vi "GetFootnoteReference.vi"(8 "error in (no error)":errorcluster, 11 "Footnote in":refnum<class "Footnote.lvclass">) -> (0 "error out":errorcluster, 2 "LvMarkdown.lvlib:FootnoteReference.lvclass":refnum<class "FootnoteReference.lvclass">, 3 "Footnote out":refnum<class "Footnote.lvclass">)   [LabVIEW 2021, in "LvMarkdown.lvlib" / "Footnote.lvclass"]
uses:
  Footnote.lvclass
  Footnote.lvclass/Footnote.ctl
  FootnoteReference/FootnoteReference.lvclass
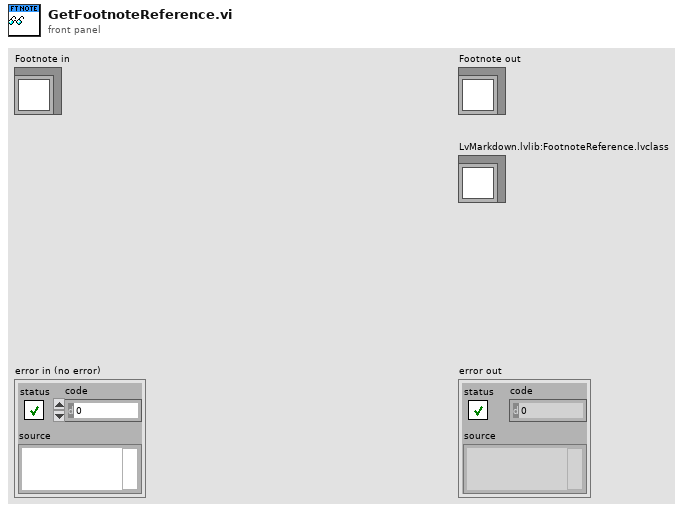
[diagram p1: front panel]
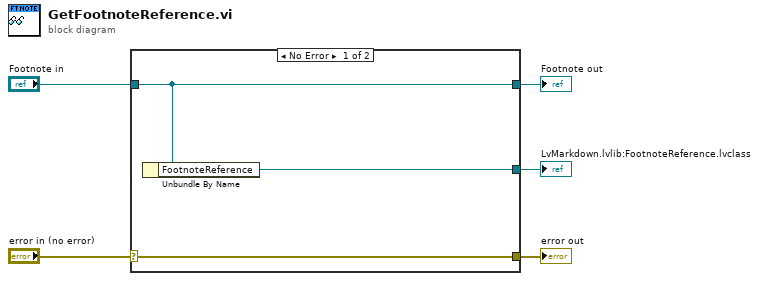
[diagram p0: block diagram]
diagram:
  n1 = case shown="No Error" "error in (no error)" {
    selector: "error in (no error)" -> [w8 w9]
    tunnel: [w8 w9] -> w4
    tunnel: [w7 w10] -> w2
    tunnel: "Footnote in" -> [w7 w10]
    tunnel: [w6 _] -> w1
    frame No Error {
      n2 = Unbundle By Name(w7) -> ("FootnoteReference"=w6:refnum<class "FootnoteReference.lvclass">)
    }
    frame Error {
    }
  }
  "error out" <- w4
  "Footnote out" <- w2
  "LvMarkdown.lvlib:FootnoteReference.lvclass" <- w1
